vi "light_sensor_filter.vi"() -> ()   [LabVIEW 2018]
panel:
  in  "timeOfMidpoint 5":fxp<+,41,40>
  in  "timeOfMidpoint 4":fxp<+,41,40>
  in  "timeOfMidpoint 3":fxp<+,41,40>
  in  "timeOfMidpoint 2":fxp<+,41,40>
  in  "timeOfMidpoint":fxp<+,41,40>
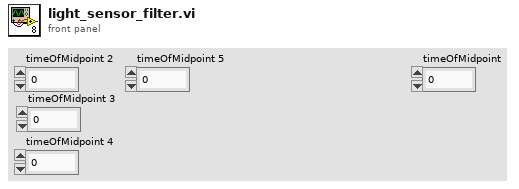
[diagram p1: front panel]
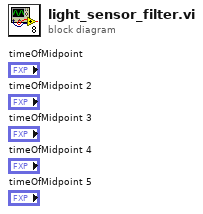
[diagram p0: block diagram]
diagram:
